vi "ILAB_CaseHandlerNoPath.vi"(2 "data":string, 3 "action":string) -> (0 "errorOut":string, 1 "response":string)   [LabVIEW 2009]
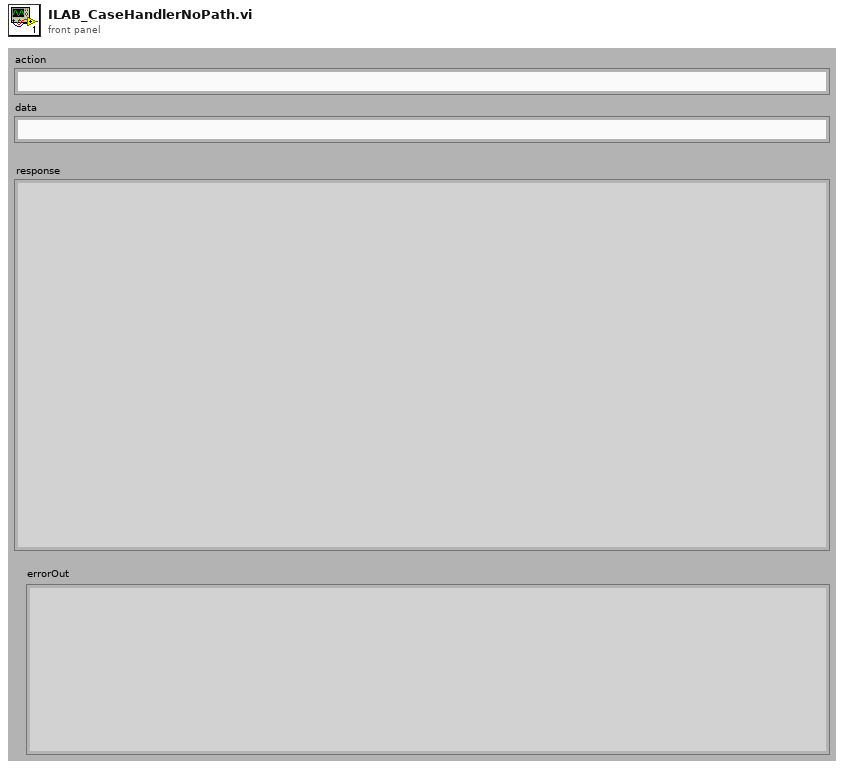
[diagram p1: front panel]
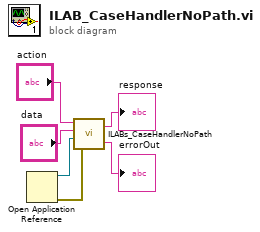
[diagram p0: block diagram]
diagram:
  n1 = Open Application Reference() -> (0:w1:errorcluster, 3:w2:refnum<vi>)  [unwired: 1 in, 3 out]
  n2 = call "ILABs_CaseHandlerNoPath.vi"("error In"=w1, "appReference"=w2, "data"="data", "action"="action") -> ("errorOut"=→"errorOut":string, "response"=→"response":string)
